vi "23384_Davis_Poku_Amankwa_Amankwa.DavisPoku.MNE1201.7.8_348263_583592853.vi"() -> ()   [LabVIEW 2018]
uses:
  <vilib>/imath/engines/lvmath2/RunTimeEngine/Managers/WorkSpace/UID Generator.vi
  <vilib>/imath/engines/lvmath2/RunTimeEngine/BuiltInFunctions/linramp/NIMS_linramp.vi
  <vilib>/imath/engines/lvmath2/RunTimeEngine/RunTimeType/NIMS_RunTimeType_From StrictType (excl LVString).vi
  <instcachedir>/0/NIMS_RunTimeType_From StrictType (excl LVString)_201635486D724C82825D35238731EDF5.lvgen/NIMS_RunTimeType_From StrictType (excl LVString)_201635486D724C82825D35238731EDF5_000.vi
  <vilib>/imath/engines/lvmath2/RunTimeEngine/LocalVariableDefStatement/MC_LocalVariableDefStatement_Display.vi
  <vilib>/imath/engines/lvmath2/RunTimeEngine/ArithmeticOperatorToken/NIMS_ArithmeticOperator_power(S).vi
  <instcachedir>/0/NIMS_ArithmeticOperator_power(S)_3478FB393A97485A9403569FA13F458B.lvgen/NIMS_ArithmeticOperator_power(S)_3478FB393A97485A9403569FA13F458B_014.vi
  <vilib>/imathl/engines/lvmath/Functions/Error Handling/Create Error.vi
  <vilib>/imath/engines/lvmath2/RunTimeEngine/Managers/SymbolTable/Clear UID.vi
  <vilib>/imath/engines/lvmath2/RunTimeEngine/NodeEndStatement/NIMS_NodeEndStatement_Output.vi
  <instcachedir>/0/NIMS_NodeEndStatement_Output_53EC0D466D134D7ABD903AC30B43404B.lvgen/NIMS_NodeEndStatement_Output_53EC0D466D134D7ABD903AC30B43404B_000.vi
  <instcachedir>/0/NIMS_NodeEndStatement_Output_53EC0D466D134D7ABD903AC30B43404B.lvgen/NIMS_NodeEndStatement_Output_53EC0D466D134D7ABD903AC30B43404B_005.vi
  <vilib>/imath/engines/lvmath2/RunTimeEngine/ErrorHandling/NIMS_Finalize Error.vi
  <vilib>/imath/engines/lvmath2/RunTimeEngine/Managers/SymbolTable/NIMS_WorkSpace.lvlib
panel:
  out "XY Graph":cluster{dbl[], dbl[]}(graph)
  in  "Bode?":bool
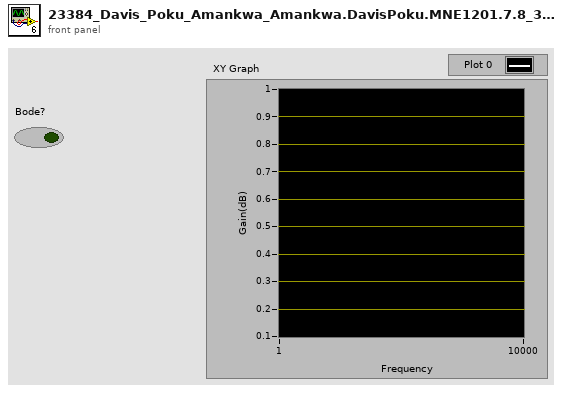
[diagram p1: front panel]
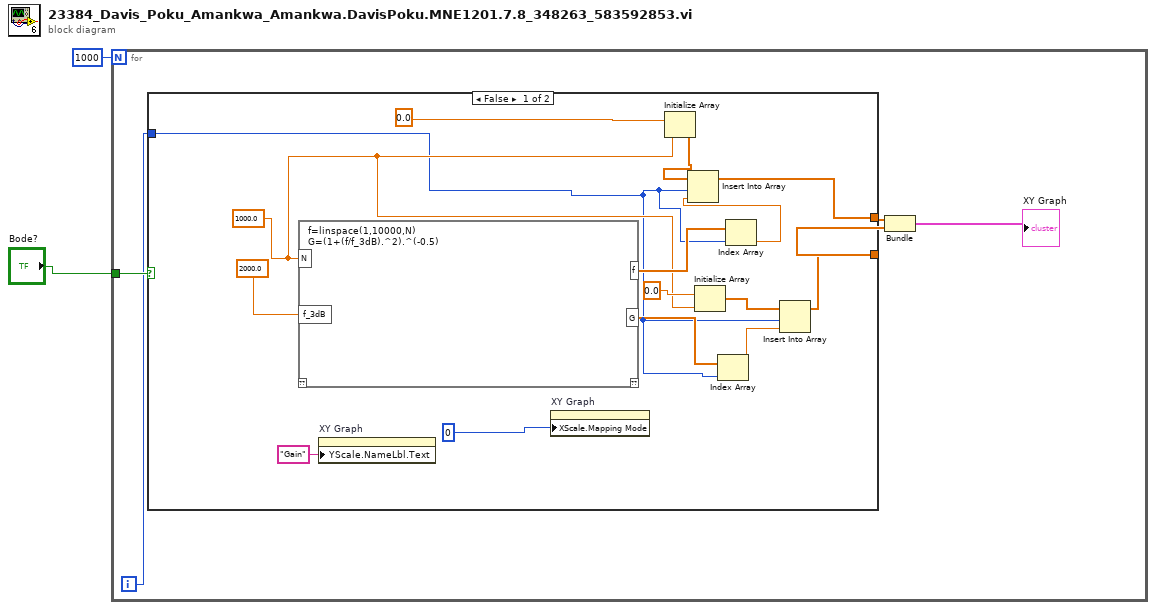
[diagram p0: block diagram]
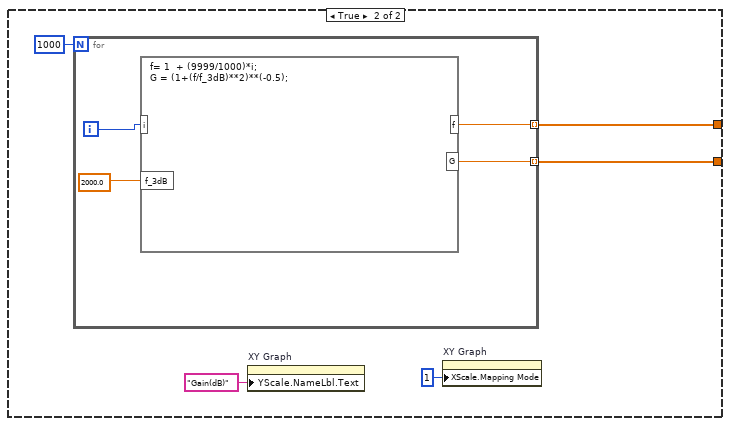
[diagram p2: hidden frame]
diagram:
  n1 = for {
    N: 1000 -> [_]
    tunnel: "Bode?" -> [w7]
    i -> [w3]
    n2 = case shown="False" w7 {
      tunnel: [w17 w99] -> w4
      tunnel: [w11 w98] -> w5
      tunnel: w3 -> [w10 _]
      frame False {
        w14 = 1000.0
        n3 = mathscript code="f=linspace(1,10000,N)\nG=(1+(f/f_3dB).^2).^(-0.5)"("N"=w14, "f_3dB"=2000.0) -> ("f"=w19:dbl[], "G"=w12:cdb[])  [unwired: 1 in, 1 out]
        n4 = property on="XY Graph" class="XYGraph (strict)"("YScale.NameLbl.Text"="Gain" ("Y Scale.Name Label.Text")) -> ()  [unwired: 2 in, 2 out]
        n5 = property on="XY Graph" class="XYGraph (strict)"("XScale.Mapping Mode"=u8 0 ("X Scale.Mapping Mode")) -> ()  [unwired: 2 in, 2 out]
        n6 = Initialize Array(0.0, w14) -> (w20:dbl[])
        n7 = Initialize Array(0.0, w14) -> (w15:dbl[])
        n8 = Index Array(array=w12, index=w10) -> (element=w13:cdb)
        n9 = Index Array(array=w19, index=w10) -> (element=w18:dbl)
        n10 = Insert Into Array(array=w20, index=w10, new element=w18) -> (w17:dbl[])
        n11 = Insert Into Array(array=w15, index=w10, new element=w13) -> (w11:dbl[])
      }
      frame True {
        n12 = for {
          N: 1000 -> [_]
          tunnel: [w102] -> w99 mode=indexing
          tunnel: [w101] -> w98 mode=indexing
          i -> [w104]
          n13 = formula code="f= 1  + (9999/1000)*i;\nG = (1+(f/f_3dB)**2)**(-0.5);"("i"=w104, "f_3dB"=2000.0) -> ("f"=w102:dbl, "G"=w101:dbl)
        }
        n14 = property on="XY Graph" class="XYGraph (strict)"("YScale.NameLbl.Text"="Gain(dB)" ("Y Scale.Name Label.Text")) -> ()  [unwired: 2 in, 2 out]
        n15 = property on="XY Graph" class="XYGraph (strict)"("XScale.Mapping Mode"=u8 1 ("X Scale.Mapping Mode")) -> ()  [unwired: 2 in, 2 out]
      }
    }
    n16 = Bundle(w4, w5) -> (→"XY Graph":cluster{dbl[], dbl[]})  [unwired: 1 in]
  }
